vi "addCaloriesToBackpack.vi"(8 "error in (no error)":errorcluster, 10 "Calories":i32, 11 "Elf in":refnum<class "Elf.lvclass">) -> (0 "error out":errorcluster, 3 "Elf out":refnum<class "Elf.lvclass">)   [LabVIEW 2017, in "Elf.lvclass"]
uses:
  Elf.lvclass
  Elf.lvclass/Elf.ctl
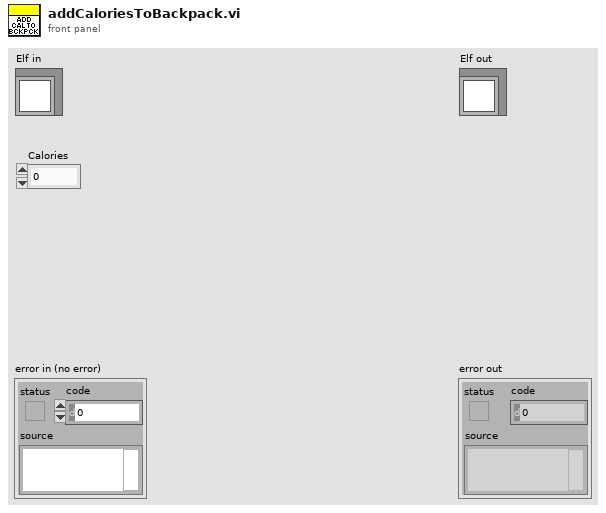
[diagram p1: front panel]
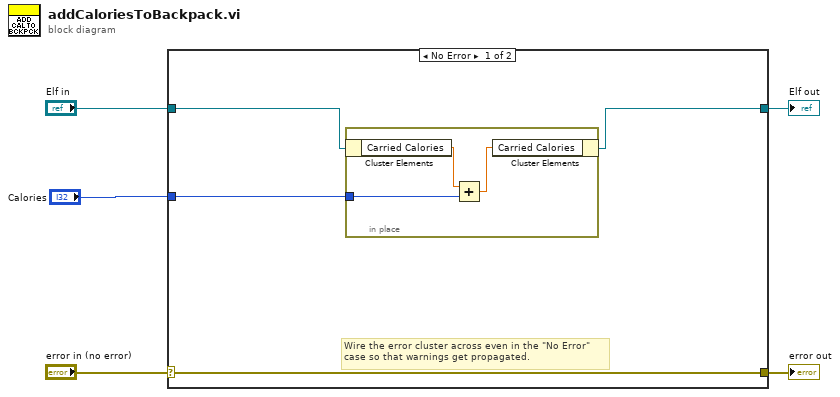
[diagram p0: block diagram]
diagram:
  n1 = case shown="No Error" "error in (no error)" {
    selector: "error in (no error)" -> [w9 w14]
    tunnel: [w9 w14] -> w4
    tunnel: [w6 w13] -> w2
    tunnel: "Elf in" -> [w7 w13]
    tunnel: "Calories" -> [w8 _]
    frame No Error {
      # "Wire the error cluster across even in the \"No Error\"\ncase so that warnings get propagated."
      n2 = in-place {
        in-place-border: w8 -> [w10]
        n3 = in-place-cluster #1(w7) -> ("Carried Calories"=w12:dbl)
        n4 = Add(x=w12, y=w10) -> (x+y=w11:dbl)
        n5 = in-place-cluster #1("Carried Calories"=w11) -> (w6:refnum<class "Elf.lvclass">)
      }
    }
    frame Error {
    }
  }
  "error out" <- w4
  "Elf out" <- w2
